vi "Main.vi"(6 "Number of Terms":dbl, 8 "stop":bool, 9 "Draw Circle?":bool, 10 "Period":dbl, 11 "Signal":cdb[](array[numeric])) -> (2 "Time":dbl, 3 "XY Graph":cluster{dbl[], dbl[]}[](graph))   [LabVIEW 2020]
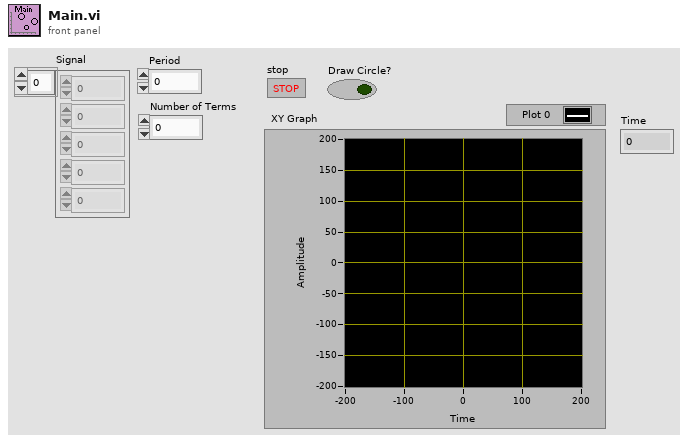
[diagram p1: front panel]
types:
  T1 = typedef "Component.ctl" = cluster{"Radius Formula":string, "Frequency":dbl, "Phase Offset":dbl}
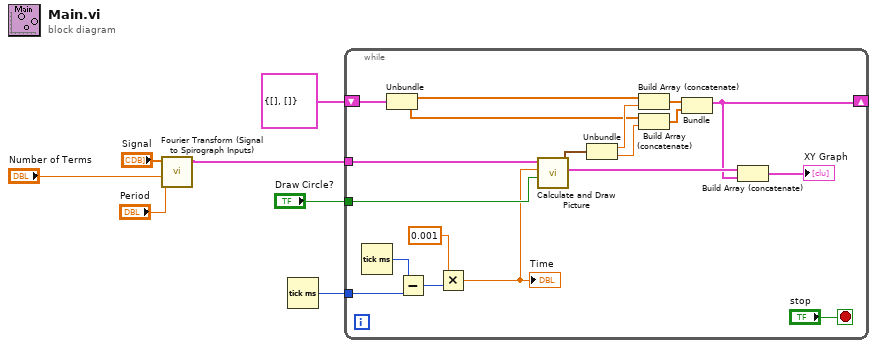
[diagram p0: block diagram]
diagram:
  n1 = call "Fourier Transform (Signal to Spirograph Inputs).vi"("Number of Terms"="Number of Terms", "Period"="Period", "Signal"="Signal") -> ("Inputs"=w4:T1[])  [unwired: 8 in]
  n2 = Tick Count (ms)() -> (millisecond timer value=w7:u32)
  n3 = while {
    tunnel: w4 -> [w23]
    tunnel: w7 -> [w26]
    tunnel: "Draw Circle?" -> [w24]
    shift-right: [w11] -> _
    shift-left: cluster{dbl[], dbl[]} {[], []} -> [w19]
    stop <- "stop" stop-if-true
    n4 = Tick Count (ms)() -> (millisecond timer value=w25:u32)
    n5 = Unbundle(w19) -> (w18:dbl[], w15:dbl[])
    n6 = Subtract(x=w25, y=w26) -> (x-y=w22:u32)
    n7 = Multiply(x=0.001, y=w22) -> (x*y=w8:dbl)
    "Time" <- w8
    n8 = call "Calculate and Draw Picture.vi"("Draw Circle?"=w24, "Time"=w8, "Inputs"=w23) -> ("Points"=w12:cluster{dbl[], dbl[]}[], "Endpoint"=w20:cluster{"x":dbl, "y":dbl})  [unwired: 7 in]
    n9 = Unbundle(w20) -> ("x"=w17:dbl, "y"=w16:dbl)
    n10 = Build Array (concatenate)(w18, w17) -> (w14:dbl[])
    n11 = Build Array (concatenate)(w15, w16) -> (w13:dbl[])
    n12 = Bundle(w14, w13) -> (w11:cluster{dbl[], dbl[]})  [unwired: 1 in]
    n13 = Build Array (concatenate)(w12, w11) -> (→"XY Graph":cluster{dbl[], dbl[]}[])
  }
